vi "Set Timeout Trigger.vi"(8 "error in (no error)":errorcluster, 10 "Trigger Settings":T1, 11 "DPO4104 in":refnum<class "DPO4104.lvclass">) -> (0 "error out":errorcluster, 3 "DPO4104 out":refnum<class "DPO4104.lvclass">)   [LabVIEW 2018, in "DPO4104.lvlib" / "DPO4104.lvclass"]
doc: "This Override is used to configure a TimeOut Trigger."
uses:
  DPO4104.lvclass
  PPLs/Oscilloscope/Parent/Oscilloscope.lvlibp/Custom Controls/Timeout Trigger Settings.ctl
  PPLs/Oscilloscope/Parent/Oscilloscope.lvlibp/Custom Controls/Analog Channels.ctl
  PPLs/Oscilloscope/Parent/Oscilloscope.lvlibp/Custom Controls/Trigger Mode.ctl
  PPLs/Oscilloscope/Parent/Oscilloscope.lvlibp/Custom Controls/Trigger Polarity.ctl
  PPLs/Oscilloscope/Parent/Oscilloscope.lvlibp/Oscilloscope.lvclass
  <instrlib>/Tektronix DPO MSO 2000 4000 Series/Tektronix DPO MSO 2000 4000 Series.lvlib
  C:/Projects/LabVIEW/PPLs/Oscilloscope/Parent/Oscilloscope.lvlibp/Oscilloscope.lvclass
  PPLs/Oscilloscope/Parent/Oscilloscope.lvlibp
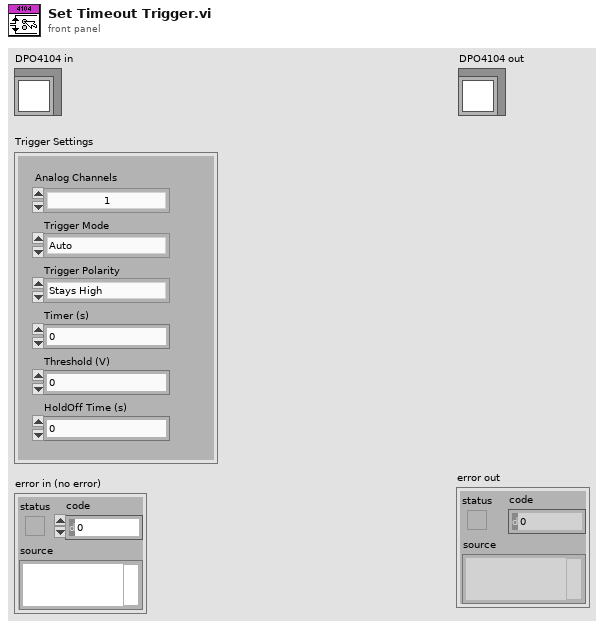
[diagram p1: front panel]
types:
  T1 = typedef "Oscilloscope.lvlibp/Timeout Trigger Settings.ctl" = cluster{"Analog Channels":T2, "Trigger Mode":T3, "Trigger Polarity":T4, "Timer (s)":dbl, "Threshold (V)":dbl, "HoldOff Time (s)":dbl}
  T2 = typedef "Oscilloscope.lvlibp/Analog Channels.ctl" = enum16{"1", "2", "3", "4", "5", "6", "7", "8", "9", "10", "11", "12", "13", "14", "15", "16"}
  T3 = typedef "Oscilloscope.lvlibp/Trigger Mode.ctl" = enum16{"Auto", "Normal"}
  T4 = typedef "Oscilloscope.lvlibp/Trigger Polarity.ctl" = enum16{"Stays High", "Stays Low", "Either"}
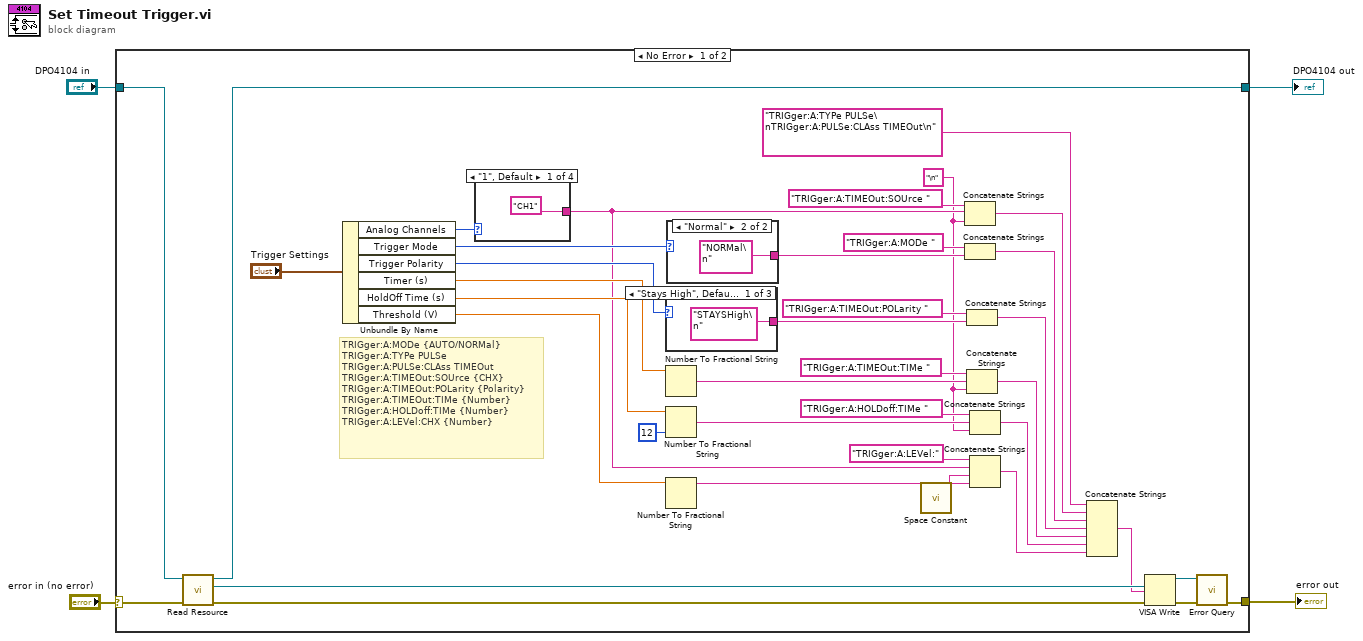
[diagram p0: block diagram]
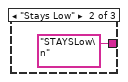
[diagram p2: hidden frame]
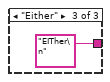
[diagram p3: hidden frame]
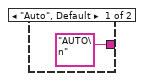
[diagram p4: hidden frame]
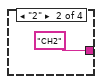
[diagram p5: hidden frame]
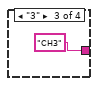
[diagram p6: hidden frame]
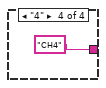
[diagram p7: hidden frame]
diagram:
  n1 = case shown="No Error" "error in (no error)" {
    selector: "error in (no error)" -> [w42 w53]
    tunnel: [w36 w53] -> w3
    tunnel: [w40 w52] -> w2
    tunnel: "DPO4104 in" -> [w41 w52]
    frame No Error {
      w7 = "\n" ("string")
      # "TRIGger:A:MODe {AUTO/NORMal}\nTRIGger:A:TYPe PULSe\nTRIGger:A:PULSe:CLAss TIMEOut\nTRIGger:A:TIMEOut:SOUrce {CHX}\nTRIGger:A:TIMEOut:POLarity {Polarity}\nTRIGger:A:TIMEOut:TIMe {Number}\nTRIGger:A:HOLDoff:TIMe {Number}\nTRIGger:A:LEVel:CHX {Number}"
      n2 = call "Read Resource.vi"("error in (no error)"=w42, "Oscilloscope in"=w41) -> ("error out"=w35:errorcluster, "Resource"=w9:refnum<visa-resource-name>, "Oscilloscope out"=w40:refnum<class "DPO4104.lvclass">)  [unwired: 7 in]
      n3 = Unbundle By Name("Trigger Settings") -> ("Analog Channels"=w34:T2, "Trigger Mode"=w31:T3, "Trigger Polarity"=w27:T4, "Timer (s)"=w26:dbl, "HoldOff Time (s)"=w23:dbl, "Threshold (V)"=w14:dbl)
      n4 = case shown="\"1\", Default" w34 {
        tunnel: ["CH1" "CH2" "CH3" "CH4"] -> w11
        frame "1", Default {
        }
        frame "2" {
        }
        frame "3" {
        }
        frame "4" {
        }
      }
      n5 = case shown="\"Stays High\", Default" w27 {
        tunnel: ["STAYSHigh\n" "STAYSLow\n" "EITher\n"] -> w29
        frame "Stays High", Default {
        }
        frame "Stays Low" {
        }
        frame "Either" {
        }
      }
      n6 = Number To Fractional String(number=w26) -> (F-format string=w24:string)  [unwired: 3 in]
      n7 = Number To Fractional String(number=w23, precision (6)=i16 12) -> (F-format string=w21:string)  [unwired: 2 in]
      n8 = Number To Fractional String(number=w14) -> (F-format string=w13:string)  [unwired: 3 in]
      n9 = case shown="\"Normal\"" w31 {
        tunnel: ["AUTO\n" "NORMal\n"] -> w32
        frame "Auto", Default {
        }
        frame "Normal" {
        }
      }
      n10 = call <vilib>:"Space Constant.vi"() -> ("String"=w12:string)
      n11 = Concatenate Strings("TRIGger:A:TIMEOut:SOUrce " ("string"), w11, w7) -> (w20:string)
      n12 = Concatenate Strings("TRIGger:A:MODe " ("string"), w32) -> (w19:string)
      n13 = Concatenate Strings("TRIGger:A:TIMEOut:POLarity " ("string"), w29) -> (w18:string)
      n14 = Concatenate Strings("TRIGger:A:TIMEOut:TIMe " ("string"), w24, w7) -> (w17:string)
      n15 = Concatenate Strings("TRIGger:A:HOLDoff:TIMe " ("string"), w21, w7) -> (w16:string)
      n16 = Concatenate Strings("TRIGger:A:LEVel:" ("string"), w11, w12, w13) -> (w10:string)
      n17 = Concatenate Strings("TRIGger:A:TYPe PULSe\nTRIGger:A:PULSe:CLAss TIMEOut\n", w20, w19, w18, w17, w16, w10) -> (w8:string)
      n18 = VISA Write(VISA resource name=w9, write buffer=w8, error in (no error)=w35) -> (VISA resource name out=w38:refnum<visa-resource-name>, error out=w37:errorcluster)  [unwired: 1 out]
      n19 = call <instrlib>:"Error Query.vi"("error in (no error)"=w37, "VISA resource name"=w38) -> ("error out"=w36:errorcluster)  [unwired: 6 in, 3 out]
    }
    frame Error {
    }
  }
  "error out" <- w3
  "DPO4104 out" <- w2
